vi "DSF.Engine.Plugin.Set Thread ID Pool.vi"(10 "Thread ID Pool":refnum<class "DSF.Engine.Pool.ID.lvclass">, 11 "Plugin in":refnum<class "DSF.Engine.Plugin.lvclass">) -> (3 "Plugin out":refnum<class "DSF.Engine.Plugin.lvclass">)   [LabVIEW 2017, in "DSF.Engine.lvlib" / "DSF.Engine.Plugin.lvclass"]
uses:
  DSF.Engine.Plugin.lvclass
  Thread Pool/DSF.Engine.Pool.ID.lvclass
  DSF.Engine.Plugin.lvclass/DSF.Engine.Plugin.ctl
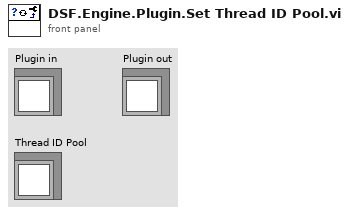
[diagram p1: front panel]
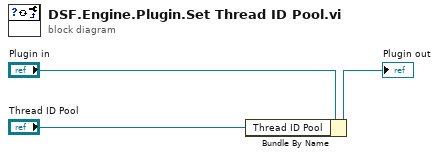
[diagram p0: block diagram]
diagram:
  n1 = Bundle By Name(cluster="Plugin in", "Thread ID Pool"="Thread ID Pool") -> (→"Plugin out":refnum<class "DSF.Engine.Plugin.lvclass">)
